vi "DutyAccelM1M2.vi"(5 "Accel1":u32 max=127 step=1, 7 "Duty1":i16 max=127 step=1, 8 "error in (no error)":errorcluster, 10 "Address":u8, 11 "VISA Refnum in":refnum<visa-resource-name>) -> (0 "error out":errorcluster, 2 "Valid":bool, 3 "VISA Refnum out":refnum<visa-resource-name>)   [LabVIEW 2015, in "Ion Motion Roboclaw.lvlib"]
uses:
  <instrlib>/Ion Motion Roboclaw/Ion Motion Roboclaw.lvlib
panel:
  in  "Accel2":u32
  in  "Duty2":i16
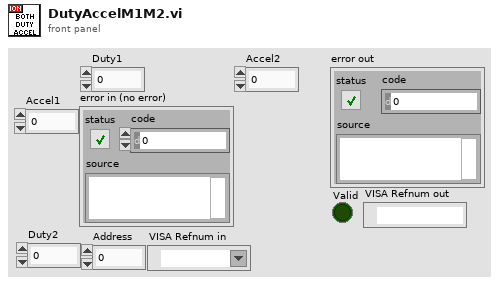
[diagram p1: front panel]
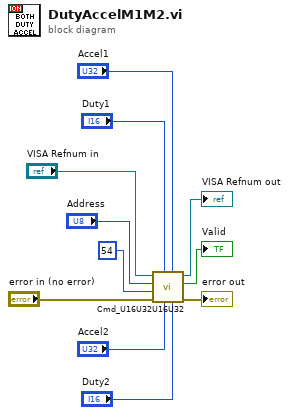
[diagram p0: block diagram]
diagram:
  n1 = call <instrlib>:"Cmd_U16U32U16U32.vi"("Arg3"="Duty2", "Arg2"="Accel1", "Arg4"="Accel2", "Arg1"="Duty1", "error in (no error)"="error in (no error)", "Cmd"=u8 54, "Address"="Address", "VISA Refnum in"="VISA Refnum in") -> ("error out"=→"error out":errorcluster, "Valid"=→"Valid":bool, "VISA Refnum out"=→"VISA Refnum out":refnum<visa-resource-name>)  [unwired: 1 in]
